vi "Advanced SCP File Download.vi"() -> ()   [LabVIEW 2018]
doc: "Downloads, or receives, any file from a remote SSH server in an efficient, iterative manner. This is similar to the SCP command line utility when transferring, or copying, a remote file to a local destination. Provides advanced functionality to monitoring and optimize performance."
uses:
  Toolkit/File Info/File Info.lvclass/File Info.ctl
  Toolkit/SSH/SSH.lvclass/SSH.ctl
  Toolkit/SSH/Utility/Read Shared Library.vi
  Toolkit/Session/Support/Password Authentication.vi
  Toolkit/File Info/Support/Create from Session.vi
  Toolkit/Channel/Support/Create from SCP Receive.vi
  Toolkit/Support/Check Status.vi
  Toolkit/File Info/Support/Destroy to Channel.vi
  Toolkit/Channel/Support/Destroy to Session.vi
  Toolkit/SSH/SSH.lvclass
  Toolkit/Session/Session.lvclass
  Toolkit/Channel/Channel.lvclass
  Toolkit/File Info/File Info.lvclass
panel:
  in  "Abort Download":bool
  out "Download Progress":dbl(slide) scale=0.0..1.0
  out "Bytes Downloaded":u64
  out "Block Download Rate":dbl format="%.3p"
  out "File Download Rate":dbl format="%.3p"
  out "File Download Time":dbl format="%<%H:%M:%S%3u>t"
  in  "Block Size":u64=30000
  in  "Remote File":string
  in  "Local File":path
  in  "Remote SSH Server":string
  in  "Password":string
  in  "Username":string
  # "Overview: Demonstrates transferring, or downloading, a remote file from a SSH server, similar to the SCP command line utility with advanced functionality\nInstructions:\n1. Enter the IP address or host name of the remote SSH server. This can be a CompactRIO (cRIO) running the National Instruments Linux Real-Time (NI Linux RT) operating system with the Enable Secure Shell Server (sshd) checkbox checked. \n2. Enter a username. If using a cRIO with a default configuration, then the username is \"admin\".\n3. Enter a password for the username. If using a cRIO with a default configuration, then the password is blank (empty).\n4. Enter the path and/or filename of the remote file to download. Typically, this is a POSIX/UNIX file path with a backslash, \"/\", use to separate directories and the default directory is the remote user's home directory, i.e. \"/home/admin\" on a default configured cRIO.\n5. Select a destination on the local computer for the transfer/download from the remote SSH server.\n6. Run this VI."
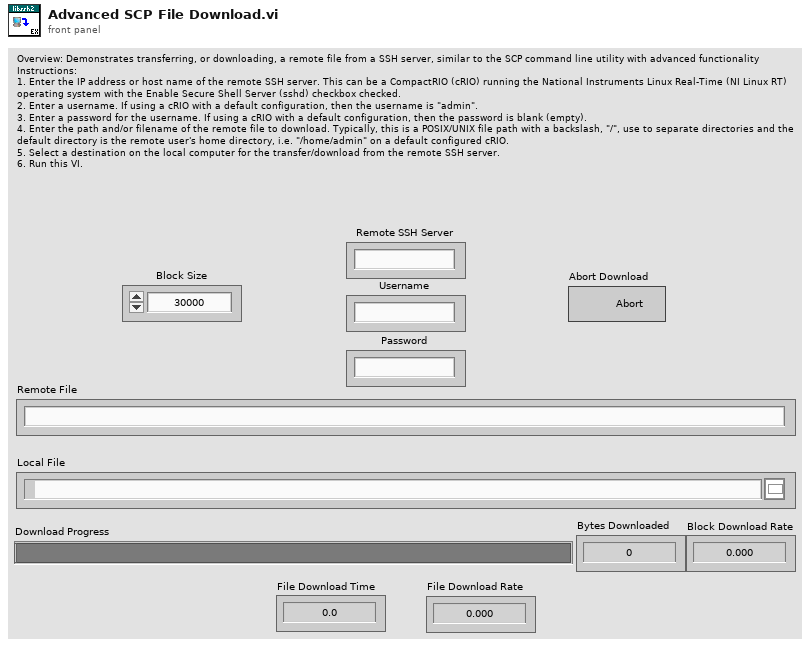
[diagram p1: front panel]
types:
  T1 = enum16{"open", "replace", "create", "open or create", "replace or create", "replace or create with confirmation"}
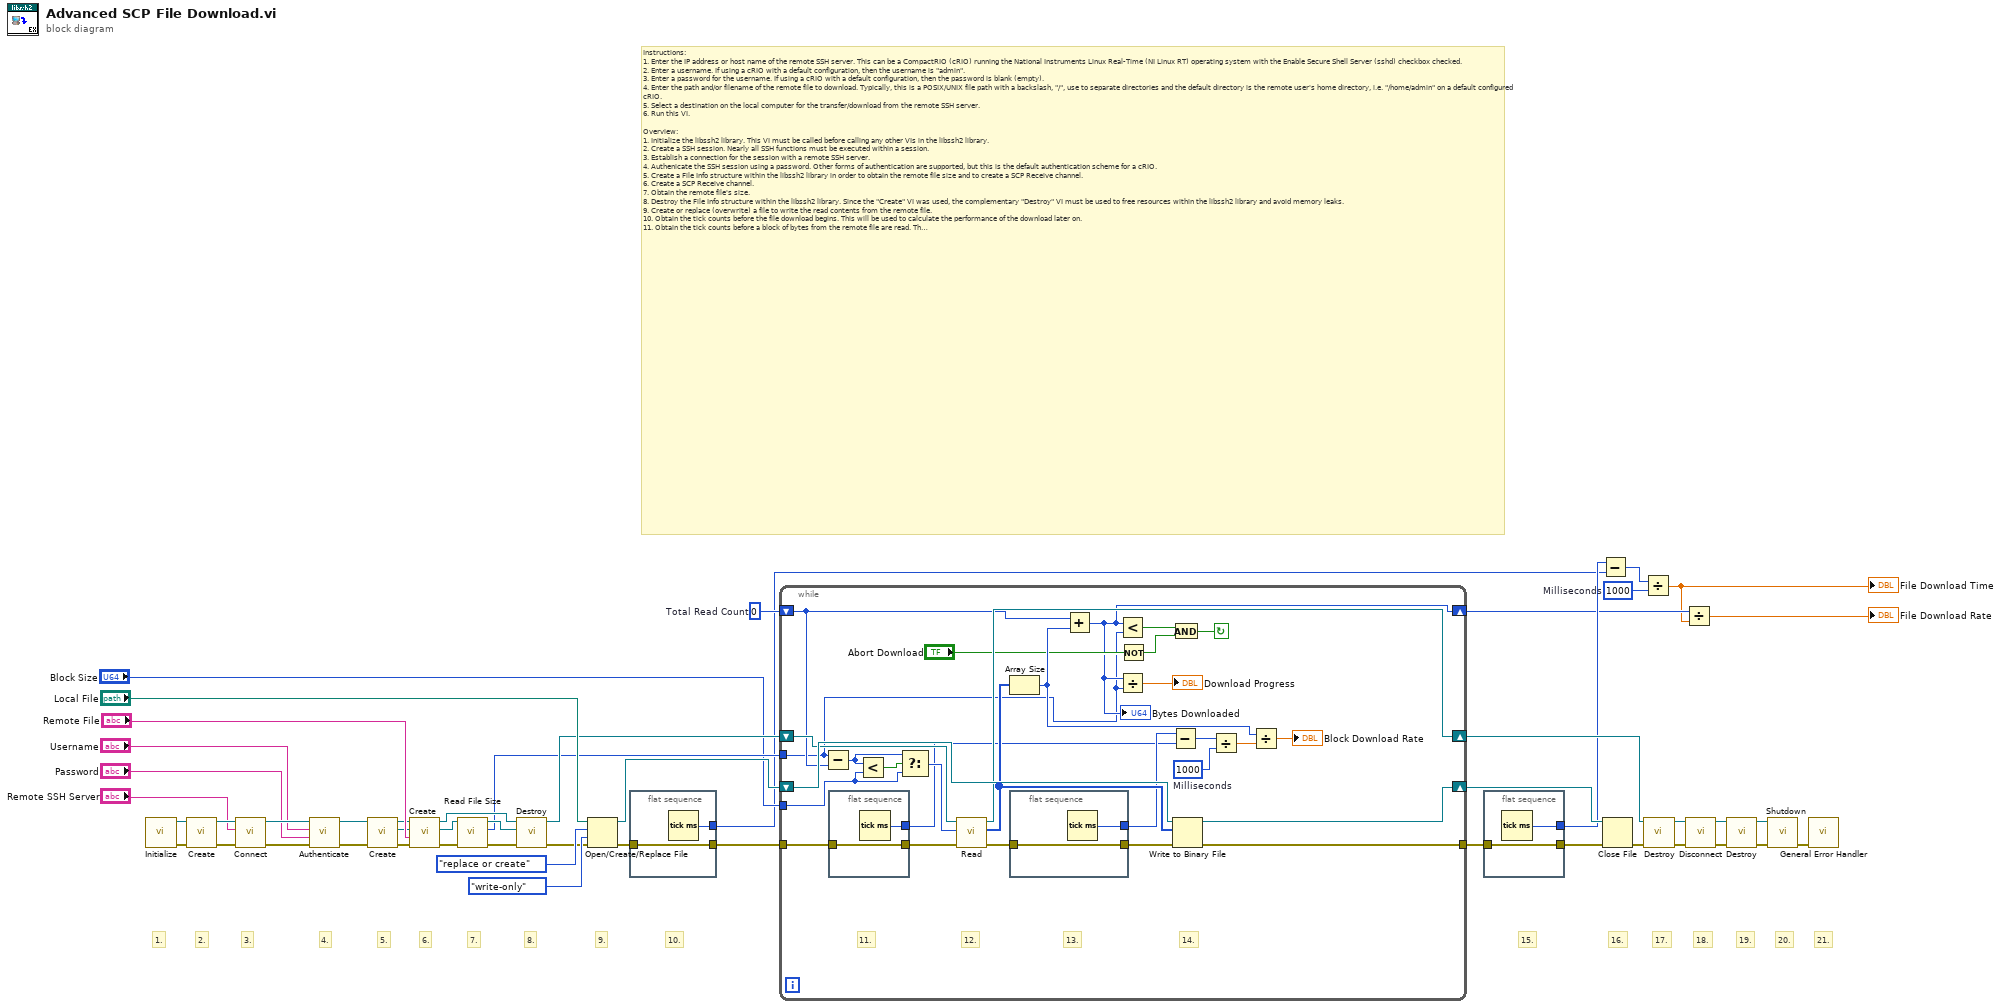
[diagram p0: block diagram]
diagram:
  w4 = u32 1000  # Milliseconds
  w14 = u64 0  # Total Read Count
  # "21."
  # "20."
  # "19."
  # "18."
  # "17."
  # "16."
  # "15."
  # "10."
  # "9."
  # "8."
  # "7."
  # "6."
  # "5."
  # "4."
  # "3."
  # "2."
  # "1."
  # "Instructions:\n1. Enter the IP address or host name of the remote SSH server. This can be a CompactRIO (cRIO) running the National Instruments Linux Real-Time (NI Linux RT) operating system with the Enable Secure Shell Server (sshd) checkbox checked. \n2. Enter a username. If using a cRIO with a default configuration, then the username is \"admin\".\n3. Enter a password for the username. If using a cRIO with a default configuration, then the password is blank (empty).\n4. Enter the path and/or filename of the remote file to download. Typically, this is a POSIX/UNIX file path with a backslash, \"/\", use to separate directories and the default directory is the remote user's home directory, i.e. \"/home/admin\" on a default configured cRIO.\n5. Select a destination on the local computer for the transfer/download from the remote SSH server.\n6. Run this VI.\n\nOverview:\n1. Initialize the libssh2 library. This VI must be called before calling any other VIs in the libssh2 library.\n2. Create a SSH session. Nearly all SSH functions must be executed within a session.\n3. Establish a connection for the session with a remote SSH server.\n4. Authenicate the SSH session using a password. Other forms of authentication are supported, but this is the default authentication scheme for a cRIO. \n5. Create a File Info structure within the libssh2 library in order to obtain the remote file size and to create a SCP Receive channel.\n6. Create a SCP Receive channel.\n7. Obtain the remote file's size.\n8. Destroy the File Info structure within the libssh2 library. Since the \"Create\" VI was used, the complementary \"Destroy\" VI must be used to free resources within the libssh2 library and avoid memory leaks.\n9. Create or replace (overwrite) a file to write the read contents from the remote file.\n10. Obtain the tick counts before the file download begins. This will be used to calculate the performance of the download later on.\n11. Obtain the tick counts before a block of bytes from the remote file are read. This will be used to calculate the block download performance.\n12. Read a block of bytes from the remote file.\n13. Obtain the tick counts after reading a single block of bytes. This is used to calculate the block download rate.\n14. Write the block of bytes from the remote file to the local file.\n15. Obtain the tick counts after the file download is done. This is used to calculate the file download time and rate.\n16. Close the file. This is not strictly necessary, but it is good practice.\n17. Destroy the SCP Receive channel. Since the \"Create\" VI is used, the complementary \"Destroy\" VI must be used to free resources within the libssh2 library.\n18. Disconnect from the remote SSH server.\n19. Destroy the session to free resources within the libssh2 library.\n20. Shutdown the libssh2 library. This VI must be last VI called for the libssh2 library. No other libssh2 VIs should be called once this VI is executed.\n21. Provide some error handling and reporting. Libssh2 errors will be in the -8100 range."
  n1 = call "Initialize.vi"() -> ("Error Out"=w36:errorcluster, "SSH"=w35:refnum<class "SSH.lvclass">)  [unwired: 10 in]
  n2 = call "Create.vi"("Error In"=w36, "SSH"=w35) -> ("Error Out"=w49:errorcluster, "Sesssion"=w50:refnum<class "Session.lvclass">)  [unwired: 8 in]
  n3 = call "Connect.vi"("Error In"=w49, "Address"="Remote SSH Server", "Session In"=w50) -> ("Error Out"=w47:errorcluster, "Sesssion Out"=w48:refnum<class "Session.lvclass">)  [unwired: 7 in]
  n4 = call-poly "Authenticate.vi"("Error In"=w47, "Password"="Password", "Username"="Username", "Session In"=w48) -> ("Error Out"=w31:errorcluster, "Sesssion Out"=w34:refnum<class "Session.lvclass">)  [unwired: 6 in]
  n5 = call-poly "Create.vi"("Error In"=w31, "Session In"=w34) -> ("Error Out"=w30:errorcluster, "File Info"=w32:refnum<class "File Info.lvclass">, "Session Out"=w33:refnum<class "Session.lvclass">)  [unwired: 7 in]
  n6 = call-poly "Create.vi"("Error In"=w30, "Remote Source Path"="Remote File", "File Info In"=w32, "Session"=w33) -> ("Error Out"=w27:errorcluster, "File Info Out"=w28:refnum<class "File Info.lvclass">, "Channel"=w29:refnum<class "Channel.lvclass">)  [unwired: 5 in]
  n7 = call "Read File Size.vi"("Error In"=w27, "File Info In"=w28) -> ("Error Out"=w25:errorcluster, "File Size"=w13:u64, "File Info Out"=w26:refnum<class "File Info.lvclass">)  [unwired: 7 in]
  n8 = call-poly "Destroy.vi"("Error In"=w25, "File Info"=w26, "Channel In"=w29) -> ("Error Out"=w21:errorcluster, "Channel Out"=w19:refnum<class "Channel.lvclass">)  [unwired: 7 in]
  n9 = Open/Create/Replace File(file path (use dialog)="Local File", error in=w21, operation (0:open)=T1."replace or create", access (0:read/write)=enum16{"read/write", "read-only", "write-only"}."write-only") -> (refnum out=w20:refnum<file>, error out=w11:errorcluster)  [unwired: 2 in, 1 out]
  n10 = flat-sequence {
    tunnel: w11 -> [w52]
    tunnel: [w52] -> w10
    tunnel: [w51] -> w6
    frame #0 {
      n11 = Tick Count (ms)() -> (millisecond timer value=w51:u32)
    }
  }
  n12 = while {
    shift-right: [w81] -> w17
    shift-left: w20 -> [w79]
    tunnel: w10 -> [w70]
    shift-right: [w77] -> w18
    shift-left: w19 -> [w78]
    tunnel: [w80] -> w9
    shift-right: [w55] -> w3
    shift-left: w14 -> [w74]
    tunnel: w13 -> [w54]
    tunnel: "Block Size" -> [w71]
    stop <- w57 continue-if-true
    w63 = u32 1000  # Milliseconds
    # "14."
    # "13."
    # "12."
    # "11."
    n13 = Subtract(x=w54, y=w74) -> (x-y=w73:u64)
    n14 = flat-sequence {
      tunnel: w70 -> [w85]
      tunnel: [w85] -> w69
      tunnel: [w84] -> w65
      frame #0 {
        n15 = Tick Count (ms)() -> (millisecond timer value=w84:u32)
      }
    }
    n16 = Less?(x=w73, y=w71) -> (x < y?=w75:bool)
    n17 = Select(t=w73, s=w75, f=w71) -> (s? t:f=w72:u64)
    n18 = call "Read.vi"("Error In"=w69, "Max Data Length"=w72, "Channel In"=w78) -> ("Error Out"=w68:errorcluster, "Data"=w76:u8[], "Channel Out"=w77:refnum<class "Channel.lvclass">)  [unwired: 6 in]
    n19 = Array Size(array=w76) -> (size(s)=w61:i32)
    n20 = flat-sequence {
      tunnel: w68 -> [w83]
      tunnel: [w83] -> w67
      tunnel: [w82] -> w66
      frame #0 {
        n21 = Tick Count (ms)() -> (millisecond timer value=w82:u32)
      }
    }
    n22 = Add(x=w74, y=w61) -> (x+y=w55:u64)
    "Bytes Downloaded" <- w55
    n23 = Less?(x=w55, y=w54) -> (x < y?=w58:bool)
    n24 = Divide(x=w55, y=w54) -> (x/y=→"Download Progress":dbl)
    n25 = Not(x="Abort Download") -> (.not. x?=w56:bool)
    n26 = Subtract(x=w66, y=w65) -> (x-y=w64:u32)
    n27 = And(x=w58, y=w56) -> (x .and. y?=w57:bool)
    n28 = Write to Binary File(file (use dialog)=w79, data=w76, error in=w67) -> (refnum out=w81:refnum<file>, error out=w80:errorcluster)  [unwired: 3 in, 1 out]
    n29 = Divide(x=w64, y=w63) -> (x/y=w62:dbl)
    n30 = Divide(x=w61, y=w62) -> (x/y=→"Block Download Rate":dbl)
  }
  n31 = flat-sequence {
    tunnel: w9 -> [w87]
    tunnel: [w87] -> w8
    tunnel: [w86] -> w7
    frame #0 {
      n32 = Tick Count (ms)() -> (millisecond timer value=w86:u32)
    }
  }
  n33 = Subtract(x=w7, y=w6) -> (x-y=w5:u32)
  n34 = Close File(refnum=w17, error in=w8) -> (error out=w16:errorcluster)  [unwired: 1 out]
  n35 = Divide(x=w5, y=w4) -> (x/y=w2:dbl)
  "File Download Time" <- w2
  n36 = call-poly "Destroy.vi"("Error In"=w16, "Channel"=w18) -> ("Error Out"=w42:errorcluster, "Session"=w43:refnum<class "Session.lvclass">)  [unwired: 8 in]
  n37 = Divide(x=w3, y=w2) -> (x/y=→"File Download Rate":dbl)
  n38 = call "Disconnect.vi"("Error In"=w42, "Session In"=w43) -> ("Error Out"=w40:errorcluster, "Sesssion Out"=w41:refnum<class "Session.lvclass">)  [unwired: 8 in]
  n39 = call "Destroy.vi"("Error In"=w40, "Session"=w41) -> ("Error Out"=w38:errorcluster, "SSH"=w39:refnum<class "SSH.lvclass">)  [unwired: 8 in]
  n40 = call "Shutdown.vi"("Error In"=w38, "SSH"=w39) -> ("Error Out"=w15:errorcluster)  [unwired: 9 in]
  n41 = call <vilib>:"General Error Handler.vi"("error in (no error)"=w15) -> ()  [unwired: 10 in, 5 out]
